vi "Test WS Connection Callback.vi"(7 "Owner":refnum<class>, 10 "Connection State":T1) -> ()   [LabVIEW 2020]
uses:
  <vilib>/IlluminatedG/lv-stream/Connection State.ctl
  <vilib>/IlluminatedG/lv-stream/Stream.lvlib
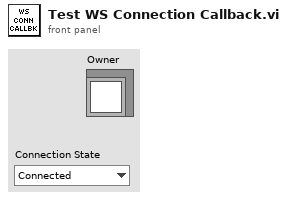
[diagram p1: front panel]
types:
  T1 = typedef "Stream.lvlib/Connection State.ctl" = enum16{"Connected", "Disconnected"}
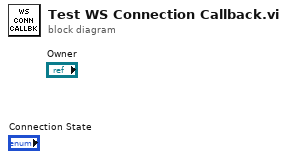
[diagram p0: block diagram]
diagram:
